vi "test Negative (Signed) BNR Parameter.vi"(8 "error in (no error)":errorcluster, 11 "TestCase in":refnum<class "Tests.lvclass">) -> (0 "error out":errorcluster, 3 "TestCase out":refnum<class "Tests.lvclass">)   [LabVIEW 2020, in "Tests.lvclass"]
uses:
  Tests.lvclass
  Parameter Definition.ctl
  Encoding and Decoding/Encoding.ctl
  32-bit Word.lvclass/32-bit Word.ctl
  32-bit Word.lvclass
  <vilib>/addons/_JKI Toolkits/VI Tester/TestCase.llb/TestCase.lvclass
  Encoding and Decoding/Encoding and Decoding.lvlib
  ARINC 429.lvclass
  C:/Program Files (x86)/National Instruments/LabVIEW 2020/vi.lib/addons/_JKI Toolkits/VI Tester/TestCase.llb/TestCase.lvclass
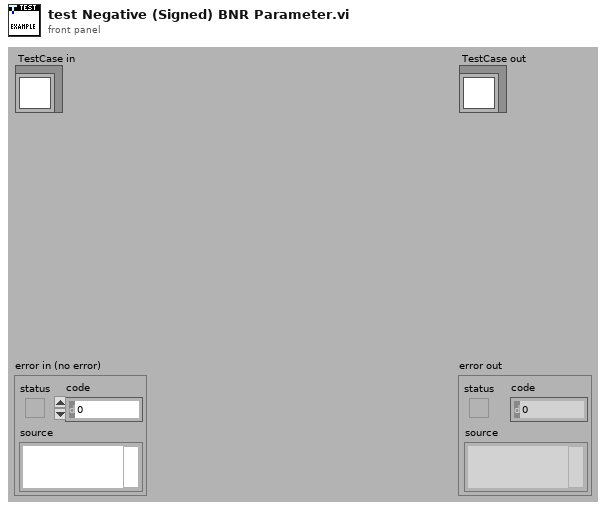
[diagram p1: front panel]
types:
  T1 = typedef "ARINC 429.lvclass/Parameter Definition.ctl" = cluster{"start index":i32, "size":i32, "encoding":T2, "signed":bool, "scale multiplier":dbl, "scale offset":dbl}
  T2 = typedef "Encoding and Decoding.lvlib/Encoding.ctl" = enum16{"BNR", "BCD", "Discrete"}
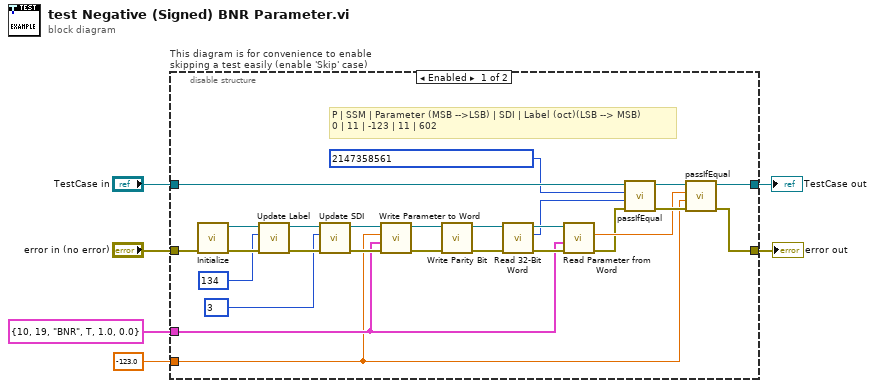
[diagram p0: block diagram]
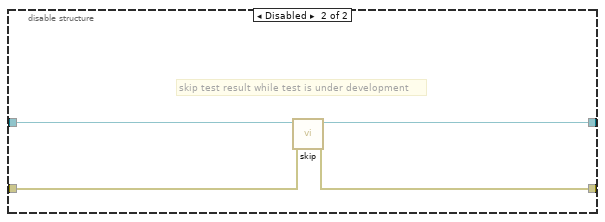
[diagram p2: hidden frame]
diagram:
  n1 = disable-structure "This diagram is for convenience to enable skipping a test easily (enable 'Skip' case)" shown="Enabled" {
    disable-tunnel: "TestCase in" -> [w13 w36]
    disable-tunnel: [w32 w34] -> w3
    disable-tunnel: [w31 w35] -> w5
    disable-tunnel: "error in (no error)" -> [w16 w33]
    disable-tunnel: T1 {"start index"=10, "size"=19, "encoding"=enum."BNR", "signed"=TRUE, "scale multiplier"=1.0, "scale offset"=0.0} ("parameter definition") -> [w9 _]
    disable-tunnel: -123.0 ("parameter value") -> [w8 _]
    frame Enabled {
      # "P | SSM | Parameter (MSB -->LSB) | SDI | Label (oct)(LSB --> MSB)\n0 | 11 | -123 | 11 | 602"
      n2 = call "Initialize.vi"("error in"=w16) -> ("error out"=w22:errorcluster, "ARINC 429 (32-bit word)"=w17:refnum<class "32-bit Word.lvclass">)  [unwired: 9 in]
      n3 = call-dynamic "Update Label.vi"("error in"=w22, "label value"=u8 134 ("label value 2"), "32-bit word in"=w17) -> ("error out"=w23:errorcluster, "32-bit word out"=w20:refnum<class "32-bit Word.lvclass">)  [unwired: 7 in]
      n4 = call-dynamic "Update SDI.vi"("error in"=w23, "SDI value"=u8 3 ("SDI value 2"), "32-bit Word in"=w20) -> ("error out"=w26:errorcluster, "32-bit Word out"=w25:refnum<class "32-bit Word.lvclass">)  [unwired: 7 in]
      n5 = call-dynamic "Write Parameter to Word.vi"("error in"=w26, "parameter definition"=w9, "data"=w8, "32-bit Word in"=w25) -> ("error out"=w27:errorcluster, "32-bit Word out"=w28:refnum<class "32-bit Word.lvclass">)  [unwired: 6 in]
      n6 = call-dynamic "Write Parity Bit.vi"("error in"=w27, "32-bit word in"=w28) -> ("error out"=w24:errorcluster, "32-bit word out"=w21:refnum<class "32-bit Word.lvclass">)  [unwired: 8 in]
      n7 = call "Read 32-Bit Word.vi"("error in (no error)"=w24, "32-bit Word in"=w21) -> ("error out"=w30:errorcluster, "32-bit word"=w11:u32, "32-bit Word out"=w29:refnum<class "32-bit Word.lvclass">)  [unwired: 7 in]
      n8 = call-dynamic "Read Parameter from Word.vi"("error in"=w30, "parameter definition"=w9, "32-bit Word in"=w29) -> ("error out"=w7:errorcluster, "parameter value"=w12:dbl)  [unwired: 6 in, 1 out]
      n9 = call-dynamic "passIfEqual.vi"("error in (no error)"=w7, "y"=w11, "x"=u32 2147358561 ("SDI value 2"), "TestCase in"=w13) -> ("error out"=w14:errorcluster, "TestCase out"=w15:refnum<class "Tests.lvclass">)  [unwired: 6 in]
      n10 = call-dynamic "passIfEqual.vi"("error in (no error)"=w14, "y"=w8, "x"=w12, "TestCase in"=w15) -> ("error out"=w31:errorcluster, "TestCase out"=w32:refnum<class "Tests.lvclass">)  [unwired: 6 in]
    }
    frame Disabled {
      # "skip test result while test is under development"
      n11 = call <vilib>:"skip.vi"("error in (no error)"=w33, "TestCase in"=w36) -> ("error out"=w35:errorcluster, "TestCase out"=w34:refnum<class "Tests.lvclass">)  [unwired: 8 in]
    }
  }
  "error out" <- w5
  "TestCase out" <- w3
